vi "LoadFilters.vi"(4 "Filter 4":u8(ring) items=["CLEAN", "B", "V", "R", "I"], 6 "Filter 3":u8(ring) items=["CLEAN", "B", "V", "R", "I"], 8 "error in (no error)":errorcluster, 9 "Filter 2":u8(ring) items=["CLEAN", "B", "V", "R", "I"], 10 "Filter 1":u8(ring) items=["CLEAN", "B", "V", "R", "I"], 11 "S4GUI in":refnum<class "S4GUI.lvclass">) -> (0 "error out":errorcluster, 3 "S4GUI out":refnum<class "S4GUI.lvclass">)   [LabVIEW 2018, in "S4GUI.lvclass"]
uses:
  S4GUI.lvclass
  S4GUI.lvclass/S4GUI.ctl
  Acquisition/Acquisition.lvclass
  Channel/Channel.lvclass
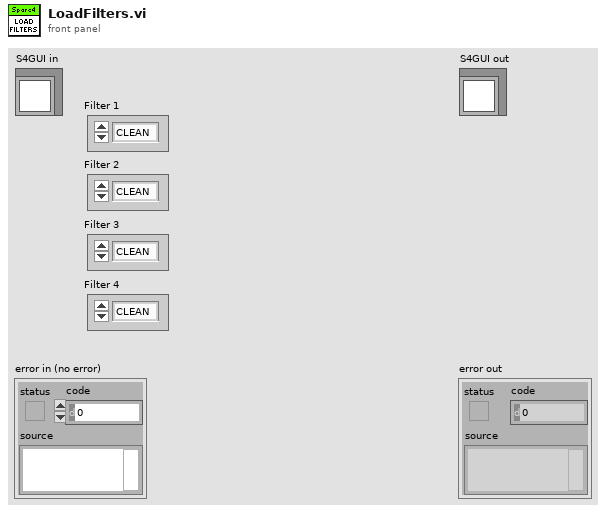
[diagram p1: front panel]
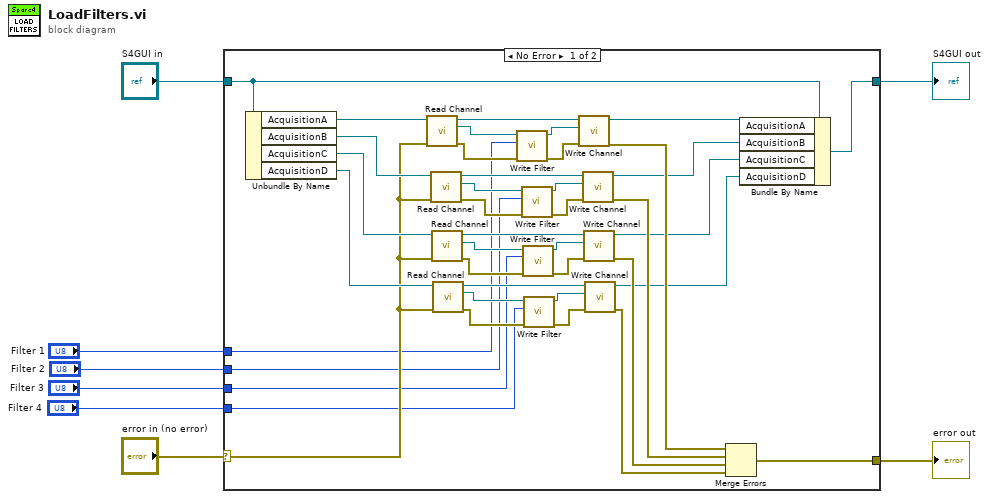
[diagram p0: block diagram]
diagram:
  n1 = case shown="No Error" "error in (no error)" {
    selector: "error in (no error)" -> [w24 w50]
    tunnel: [w19 w50] -> w7
    tunnel: [w17 w49] -> w5
    tunnel: "S4GUI in" -> [w18 w49]
    tunnel: "Filter 1" -> [w12 _]
    tunnel: "Filter 2" -> [w11 _]
    tunnel: "Filter 3" -> [w10 _]
    tunnel: "Filter 4" -> [w9 _]
    frame No Error {
      n2 = Unbundle By Name(w18) -> ("AcquisitionA"=w28:refnum<class "Acquisition.lvclass">, "AcquisitionB"=w27:refnum<class "Acquisition.lvclass">, "AcquisitionC"=w26:refnum<class "Acquisition.lvclass">, "AcquisitionD"=w25:refnum<class "Acquisition.lvclass">)
      n3 = call-dynamic "Read Channel.vi"("error in (no error)"=w24, "Acquisition in"=w28) -> ("error out"=w47:errorcluster, "Channel.lvclass"=w45:refnum<class "Channel.lvclass">, "Acquisition out"=w48:refnum<class "Acquisition.lvclass">)  [unwired: 7 in]
      n4 = call-dynamic "Read Channel.vi"("error in (no error)"=w24, "Acquisition in"=w27) -> ("error out"=w42:errorcluster, "Channel.lvclass"=w40:refnum<class "Channel.lvclass">, "Acquisition out"=w43:refnum<class "Acquisition.lvclass">)  [unwired: 7 in]
      n5 = call-dynamic "Read Channel.vi"("error in (no error)"=w24, "Acquisition in"=w26) -> ("error out"=w37:errorcluster, "Channel.lvclass"=w35:refnum<class "Channel.lvclass">, "Acquisition out"=w38:refnum<class "Acquisition.lvclass">)  [unwired: 7 in]
      n6 = call-dynamic "Read Channel.vi"("error in (no error)"=w24, "Acquisition in"=w25) -> ("error out"=w32:errorcluster, "Channel.lvclass"=w30:refnum<class "Channel.lvclass">, "Acquisition out"=w33:refnum<class "Acquisition.lvclass">)  [unwired: 7 in]
      n7 = call-dynamic "Write Filter.vi"("error in (no error)"=w47, "Filter"=w12, "Channel in"=w45) -> ("error out"=w46:errorcluster, "Channel out"=w44:refnum<class "Channel.lvclass">)  [unwired: 7 in]
      n8 = call-dynamic "Write Filter.vi"("error in (no error)"=w42, "Filter"=w11, "Channel in"=w40) -> ("error out"=w41:errorcluster, "Channel out"=w39:refnum<class "Channel.lvclass">)  [unwired: 7 in]
      n9 = call-dynamic "Write Filter.vi"("error in (no error)"=w37, "Filter"=w10, "Channel in"=w35) -> ("error out"=w36:errorcluster, "Channel out"=w34:refnum<class "Channel.lvclass">)  [unwired: 7 in]
      n10 = call-dynamic "Write Filter.vi"("error in (no error)"=w32, "Filter"=w9, "Channel in"=w30) -> ("error out"=w31:errorcluster, "Channel out"=w29:refnum<class "Channel.lvclass">)  [unwired: 7 in]
      n11 = call-dynamic "Write Channel.vi"("error in (no error)"=w46, "Channel.lvclass"=w44, "Acquisition in"=w48) -> ("error out"=w23:errorcluster, "Acquisition out"=w16:refnum<class "Acquisition.lvclass">)  [unwired: 7 in]
      n12 = call-dynamic "Write Channel.vi"("error in (no error)"=w41, "Channel.lvclass"=w39, "Acquisition in"=w43) -> ("error out"=w22:errorcluster, "Acquisition out"=w15:refnum<class "Acquisition.lvclass">)  [unwired: 7 in]
      n13 = call-dynamic "Write Channel.vi"("error in (no error)"=w36, "Channel.lvclass"=w34, "Acquisition in"=w38) -> ("error out"=w21:errorcluster, "Acquisition out"=w14:refnum<class "Acquisition.lvclass">)  [unwired: 7 in]
      n14 = call-dynamic "Write Channel.vi"("error in (no error)"=w31, "Channel.lvclass"=w29, "Acquisition in"=w33) -> ("error out"=w20:errorcluster, "Acquisition out"=w13:refnum<class "Acquisition.lvclass">)  [unwired: 7 in]
      n15 = Merge Errors(w23, w22, w21, w20) -> (w19:errorcluster)
      n16 = Bundle By Name(cluster=w18, "AcquisitionA"=w16, "AcquisitionB"=w15, "AcquisitionC"=w14, "AcquisitionD"=w13) -> (w17:refnum<class "S4GUI.lvclass">)
    }
    frame Error {
    }
  }
  "error out" <- w7
  "S4GUI out" <- w5
